vi "Untitled 3.vi"() -> ()   [LabVIEW 2017]
uses:
  <vilib>/regexp/Match Regular Expression.xnode
panel:
  out "substring":string
  out "outp":string[](array[string])
  in  "string":string
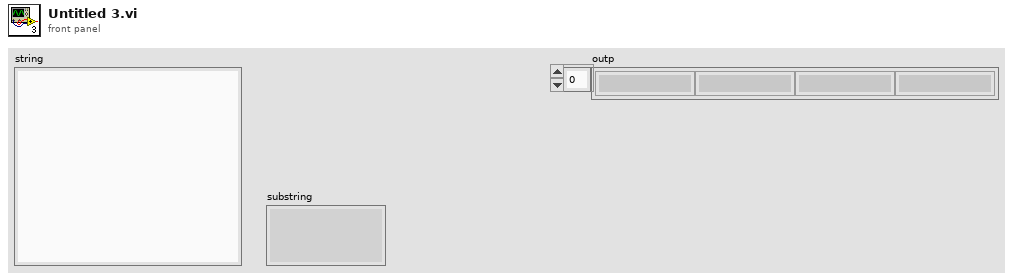
[diagram p1: front panel]
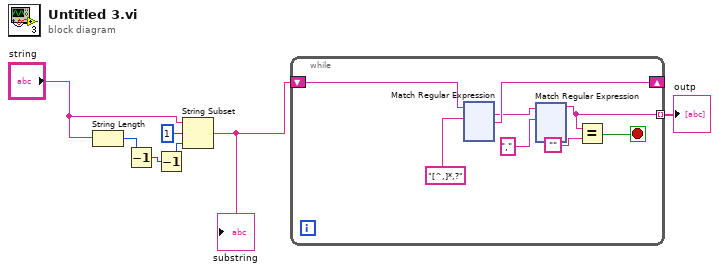
[diagram p0: block diagram]
diagram:
  n1 = String Length(string="string") -> (length=w5:i32)
  n2 = Decrement(x=w5) -> (x-1=w4:i32)
  n3 = Decrement(x=w4) -> (x-1=w3:i32)
  n4 = String Subset(string="string", offset (0)=1, length (rest)=w3) -> (substring=w1:string)
  "substring" <- w1
  n5 = while {
    tunnel: [w10] -> w7 mode=indexing
    shift-right: [w13] -> _
    shift-left: w1 -> [w14]
    stop <- w11 stop-if-true
    n6 = xnode "Match Regular Expression"("input string"=w14, "regular expression"="[^,]*,?") -> ("whole match"=w9:string, "after match"=w13:string)  [unwired: 4 in, 3 out]
    n7 = xnode "Match Regular Expression"("input string"=w9, "regular expression"=",") -> ("before match"=w10:string)  [unwired: 4 in, 4 out]
    n8 = Equal?(x=w10, y="") -> (x = y?=w11:bool)
  }
  "outp" <- w7
